vi "Retrieve Connection List.vi"(8 "error in (no error)":errorcluster, 10 "Connection List":refnum<class "Message Enqueuer.lvclass">[](array[class]), 11 "Connection Listener in":refnum<class "Connection Listener.lvclass">) -> (0 "error out":errorcluster, 3 "Connection Listener out":refnum<class "Connection Listener.lvclass">)   [LabVIEW 2017]
uses:
  Connection Listener.lvclass
  <vilib>/ActorFramework/Message Enqueuer/Message Enqueuer.lvclass
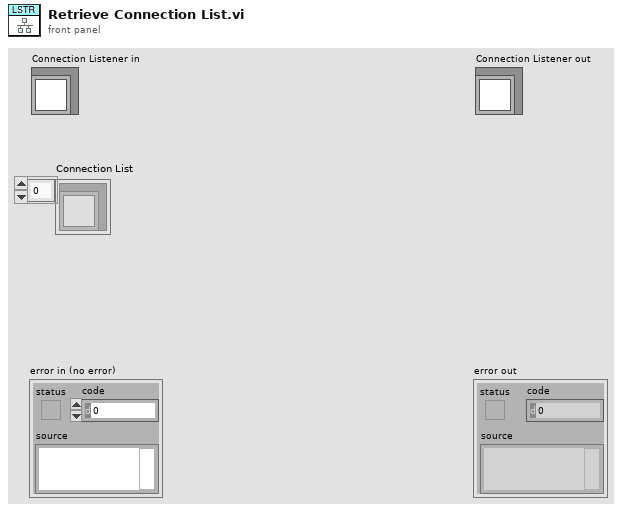
[diagram p1: front panel]
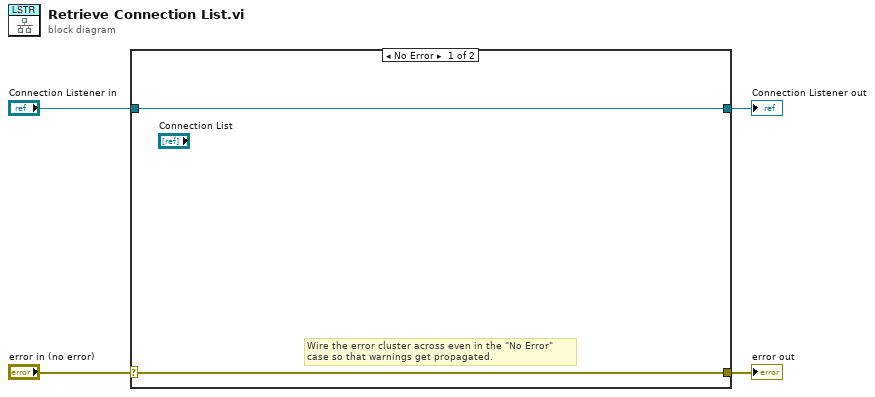
[diagram p0: block diagram]
diagram:
  n1 = case shown="No Error" "error in (no error)" {
    selector: "error in (no error)" -> [w5 w8]
    tunnel: [w5 w8] -> w3
    tunnel: [w6 w7] -> w1
    tunnel: "Connection Listener in" -> [w6 w7]
    frame No Error {
      # "Wire the error cluster across even in the \"No Error\"\ncase so that warnings get propagated."
    }
    frame Error {
    }
  }
  "error out" <- w3
  "Connection Listener out" <- w1
